vi "Kinect_posicao.vi"(11 "dado":dbl) -> (3 "Old Value":dbl)   [LabVIEW 2016]
panel:
  out "dado 3":dbl
  out "dado 2":dbl
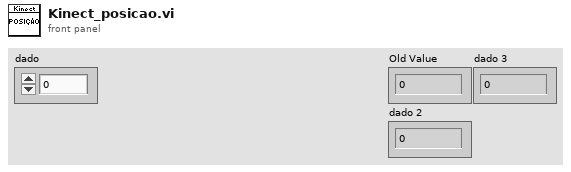
[diagram p1: front panel]
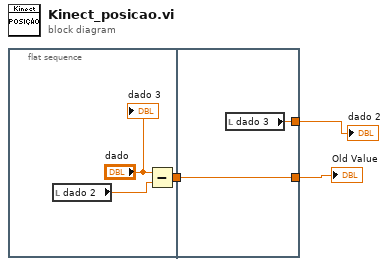
[diagram p0: block diagram]
diagram:
  n1 = flat-sequence {
    tunnel: [w5] -> w2
    tunnel: [w8] -> w3
    tunnel: w2 -> [w8]
    tunnel: [w7] -> w1
    frame #0 {
      n2 = local read "dado 2"() -> (w4:dbl)
      n3 = Subtract(x="dado", y=w4) -> (x-y=w5:dbl)
      "dado 3" <- "dado"
    }
    frame #1 {
      n4 = local read "dado 3"() -> (w7:dbl)
    }
  }
  "Old Value" <- w3
  "dado 2" <- w1
